vi "UI_(05A)_Set_Stop_State.vi"(3 "error in (no error)":errorcluster, 4 "Settings cluster in":T1={"Defaults"={"Default User"=0.0, "VISA Resource Name "=""}, "Recording and saving"={"Researcher name"="", "Name prefix"="", "Data post-processing"={"Filter type"=enum."Savitzky-Golay", "Length"=31, "Order"=3}, "Stop at"=0.0, "\"Stop at\" enabled"=FALSE, "Default save folder path"=path "", "Acquisition FPS"=enum."Max"}, "Geometry"={"Cage diameter, mm"=0, "Starting angle MIDFIELD"=0, "Starting angle BORDER"=0, "Radius, mm CENTER"=0, "Radius, mm MIDFIELD"=0, "N segments MIDFIELD"=0, "N segments BORDER"=0, "R-gap, mm"=0.0, "Bridge swap"=FALSE, "Bridge H. offset"=0.0, "Bridge V. offset"=0.0, "Twisted neck"=FALSE, "Alt. magn. orientation"=FALSE}, "IO parameters"={"IO general config."=0, "IO 1 configuration"=0, "IO 2 configuration"=0, "IO 3 configuration"=0, "IO 4 configuration"=0, "Activate ext. RS-232"=0, "IO inversion config."=0, "Sync capability"=1}, "Stimulus presets array"=[{"Event type"=0, "Dur., s"=0.0, "Stim., s"=0.0, "TTL out N"=1, "Set/Clear"=FALSE, "Stim. has been set"=FALSE}, {"Event type"=0, "Dur., s"=0.0, "Stim., s"=0.0, "TTL out N"=1, "Set/Clear"=FALSE, "Stim. has been set"=FALSE}, {"Event type"=0, "Dur., s"=0.0, "Stim., s"=0.0, "TTL out N"=1, "Set/Clear"=FALSE, "Stim. has been set"=FALSE}, {"Event type"=0, "Dur., s"=0.0, "Stim., s"=0.0, "TTL out N"=1, "Set/Clear"=FALSE, "Stim. has been set"=FALSE}, {"Event type"=0, "Dur., s"=0.0, "Stim., s"=0.0, "TTL out N"=1, "Set/Clear"=FALSE, "Stim. has been set"=FALSE}, {"Event type"=0, "Dur., s"=0.0, "Stim., s"=0.0, "TTL out N"=1, "Set/Clear"=FALSE, "Stim. has been set"=FALSE}, {"Event type"=0, "Dur., s"=0.0, "Stim., s"=0.0, "TTL out N"=1, "Set/Clear"=FALSE, "Stim. has been set"=FALSE}, {"Event type"=0, "Dur., s"=0.0, "Stim., s"=0.0, "TTL out N"=1, "Set/Clear"=FALSE, "Stim. has been set"=FALSE}, {"Event type"=0, "Dur., s"=0.0, "Stim., s"=0.0, "TTL out N"=1, "Set/Clear"=FALSE, "Stim. has been set"=FALSE}, {"Event type"=0, "Dur., s"=0.0, "Stim., s"=0.0, "TTL out N"=1, "Set/Clear"=FALSE, "Stim. has been set"=FALSE}, {"Event type"=0, "Dur., s"=0.0, "Stim., s"=0.0, "TTL out N"=1, "Set/Clear"=FALSE, "Stim. has been set"=FALSE}, {"Event type"=0, "Dur., s"=0.0, "Stim., s"=0.0, "TTL out N"=1, "Set/Clear"=FALSE, "Stim. has been set"=FALSE}, {"Event type"=0, "Dur., s"=0.0, "Stim., s"=0.0, "TTL out N"=1, "Set/Clear"=FALSE, "Stim. has been set"=FALSE}, {"Event type"=0, "Dur., s"=0.0, "Stim., s"=0.0, "TTL out N"=1, "Set/Clear"=FALSE, "Stim. has been set"=FALSE}], "Calibration parameters"={"Timing calibration sw/hw"=1.0, "True FPS"=80.0, "True frame time, s"=80.0, "Disp. calibration info"=[]}, "Settings loaded OK"=FALSE} {"Calibration parameters"."True frame time, s" format="%.10g"; "Calibration parameters"."Disp. calibration info"."Speed, µl per ms" format="%.3g"; "Calibration parameters"."True FPS" format="%.10g"; "Calibration parameters"."Timing calibration sw/hw" format="%.10g"; "Stimulus presets array"."Event type" items=["Stay for N seconds"]; "Stimulus presets array"."TTL out N" items=["1"=1, "2"=2, "1+2"=3]; "Recording and saving"."Data post-processing"."Order" min=3 max=11 step=2; "Recording and saving"."Data post-processing"."Length" min=5 max=301 step=2; "Geometry"."Cage diameter, mm" scale=0.0..340.0}, 5 "All references in":T11) -> (0 "error out":errorcluster, 1 "Settings cluster out":T1={"Defaults"={"Default User"=0.0, "VISA Resource Name "=""}, "Recording and saving"={"Researcher name"="", "Name prefix"="", "Data post-processing"={"Filter type"=enum."Savitzky-Golay", "Length"=31, "Order"=3}, "Stop at"=0.0, "\"Stop at\" enabled"=FALSE, "Default save folder path"=path "", "Acquisition FPS"=enum."Max"}, "Geometry"={"Cage diameter, mm"=0, "Starting angle MIDFIELD"=0, "Starting angle BORDER"=0, "Radius, mm CENTER"=0, "Radius, mm MIDFIELD"=0, "N segments MIDFIELD"=0, "N segments BORDER"=0, "R-gap, mm"=0.0, "Bridge swap"=FALSE, "Bridge H. offset"=0.0, "Bridge V. offset"=0.0, "Twisted neck"=FALSE, "Alt. magn. orientation"=FALSE}, "IO parameters"={"IO general config."=0, "IO 1 configuration"=0, "IO 2 configuration"=0, "IO 3 configuration"=0, "IO 4 configuration"=0, "Activate ext. RS-232"=0, "IO inversion config."=0, "Sync capability"=1}, "Stimulus presets array"=[{"Event type"=0, "Dur., s"=0.0, "Stim., s"=0.0, "TTL out N"=1, "Set/Clear"=FALSE, "Stim. has been set"=FALSE}, {"Event type"=0, "Dur., s"=0.0, "Stim., s"=0.0, "TTL out N"=1, "Set/Clear"=FALSE, "Stim. has been set"=FALSE}, {"Event type"=0, "Dur., s"=0.0, "Stim., s"=0.0, "TTL out N"=1, "Set/Clear"=FALSE, "Stim. has been set"=FALSE}, {"Event type"=0, "Dur., s"=0.0, "Stim., s"=0.0, "TTL out N"=1, "Set/Clear"=FALSE, "Stim. has been set"=FALSE}, {"Event type"=0, "Dur., s"=0.0, "Stim., s"=0.0, "TTL out N"=1, "Set/Clear"=FALSE, "Stim. has been set"=FALSE}, {"Event type"=0, "Dur., s"=0.0, "Stim., s"=0.0, "TTL out N"=1, "Set/Clear"=FALSE, "Stim. has been set"=FALSE}, {"Event type"=0, "Dur., s"=0.0, "Stim., s"=0.0, "TTL out N"=1, "Set/Clear"=FALSE, "Stim. has been set"=FALSE}, {"Event type"=0, "Dur., s"=0.0, "Stim., s"=0.0, "TTL out N"=1, "Set/Clear"=FALSE, "Stim. has been set"=FALSE}, {"Event type"=0, "Dur., s"=0.0, "Stim., s"=0.0, "TTL out N"=1, "Set/Clear"=FALSE, "Stim. has been set"=FALSE}, {"Event type"=0, "Dur., s"=0.0, "Stim., s"=0.0, "TTL out N"=1, "Set/Clear"=FALSE, "Stim. has been set"=FALSE}, {"Event type"=0, "Dur., s"=0.0, "Stim., s"=0.0, "TTL out N"=1, "Set/Clear"=FALSE, "Stim. has been set"=FALSE}, {"Event type"=0, "Dur., s"=0.0, "Stim., s"=0.0, "TTL out N"=1, "Set/Clear"=FALSE, "Stim. has been set"=FALSE}, {"Event type"=0, "Dur., s"=0.0, "Stim., s"=0.0, "TTL out N"=1, "Set/Clear"=FALSE, "Stim. has been set"=FALSE}, {"Event type"=0, "Dur., s"=0.0, "Stim., s"=0.0, "TTL out N"=1, "Set/Clear"=FALSE, "Stim. has been set"=FALSE}], "Calibration parameters"={"Timing calibration sw/hw"=1.0, "True FPS"=80.0, "True frame time, s"=80.0, "Disp. calibration info"=[]}, "Settings loaded OK"=FALSE} {"Calibration parameters"."True frame time, s" format="%.10g"; "Calibration parameters"."Disp. calibration info"."Speed, µl per ms" format="%.3g"; "Calibration parameters"."True FPS" format="%.10g"; "Calibration parameters"."Timing calibration sw/hw" format="%.10g"; "Stimulus presets array"."Event type" items=["Stay for N seconds"]; "Stimulus presets array"."TTL out N" items=["1"=1, "2"=2, "1+2"=3]; "Recording and saving"."Data post-processing"."Order" min=3 max=11 step=2; "Recording and saving"."Data post-processing"."Length" min=5 max=301 step=2; "Geometry"."Cage diameter, mm" scale=0.0..340.0}, 2 "All references out":T11)   [LabVIEW 2018, in "Tracker.lvlib"]
uses:
  Controls/CTL_All_References.ctl
  Controls/CTL_Controls_References.ctl
  Controls/CTL_Indicators_References.ctl
  Controls/CTL_Panes_and_VIs_References.ctl
  Controls/CTL_Histogram_Properties.ctl
  <vilib>/Utility/miscctls.llb/LVRangeTypeDef.ctl
  Controls/CTL_Settings_cluster.ctl
  Controls/CTL_Filter_selector.ctl
  Controls/CTL_Acquisition_speed_selector.ctl
  Controls/CTL_Segmented_plot_parameters.ctl
  Controls/CTL_IO_params_cluster.ctl
  Controls/CTL_Single_stimulus_setting.ctl
  Controls/CTL_Calibration_parameters.ctl
  Controls/CTL_Dispenser_calibration_info.ctl
  <vilib>/Utility/error.llb/Error Cluster From Error Code.vi
  <vilib>/ErrorRing/Error Ring.xnode
  Tracker.lvlib
panel:
  in  "Histogram initialization cluster":T9={"X Scale.Range"={"Minimum"=0.0, "Maximum"=13.0, "Increment"=1.0, "Minor Increment"=1.0, "Start"=0.0}, "Caption.Text"="Zone preference (normalized)", "X Scale.Offset and Multiplier:Multiplier"=1.0, "X Scale.Offset and Multiplier:Offset"=0.0, "X Scale.Scale Fit"=2, "X Scale.Display Format:Precision"=0, "Y Scale.Mapping Mode"=0, "Zones preference empty initialized array"=[0, 0, 0, 0, 0, 0, 0, 0, 0, 0, 0, 0, 0, 0], "Plot.Fill/Point Color"=15790320}
  out "Panes references":T14
  out "Controls references params":string[][](array[string])
  out "Indicators references params":string[][](array[string])
  out "Indicators references":T13
  out "Controls references":T12
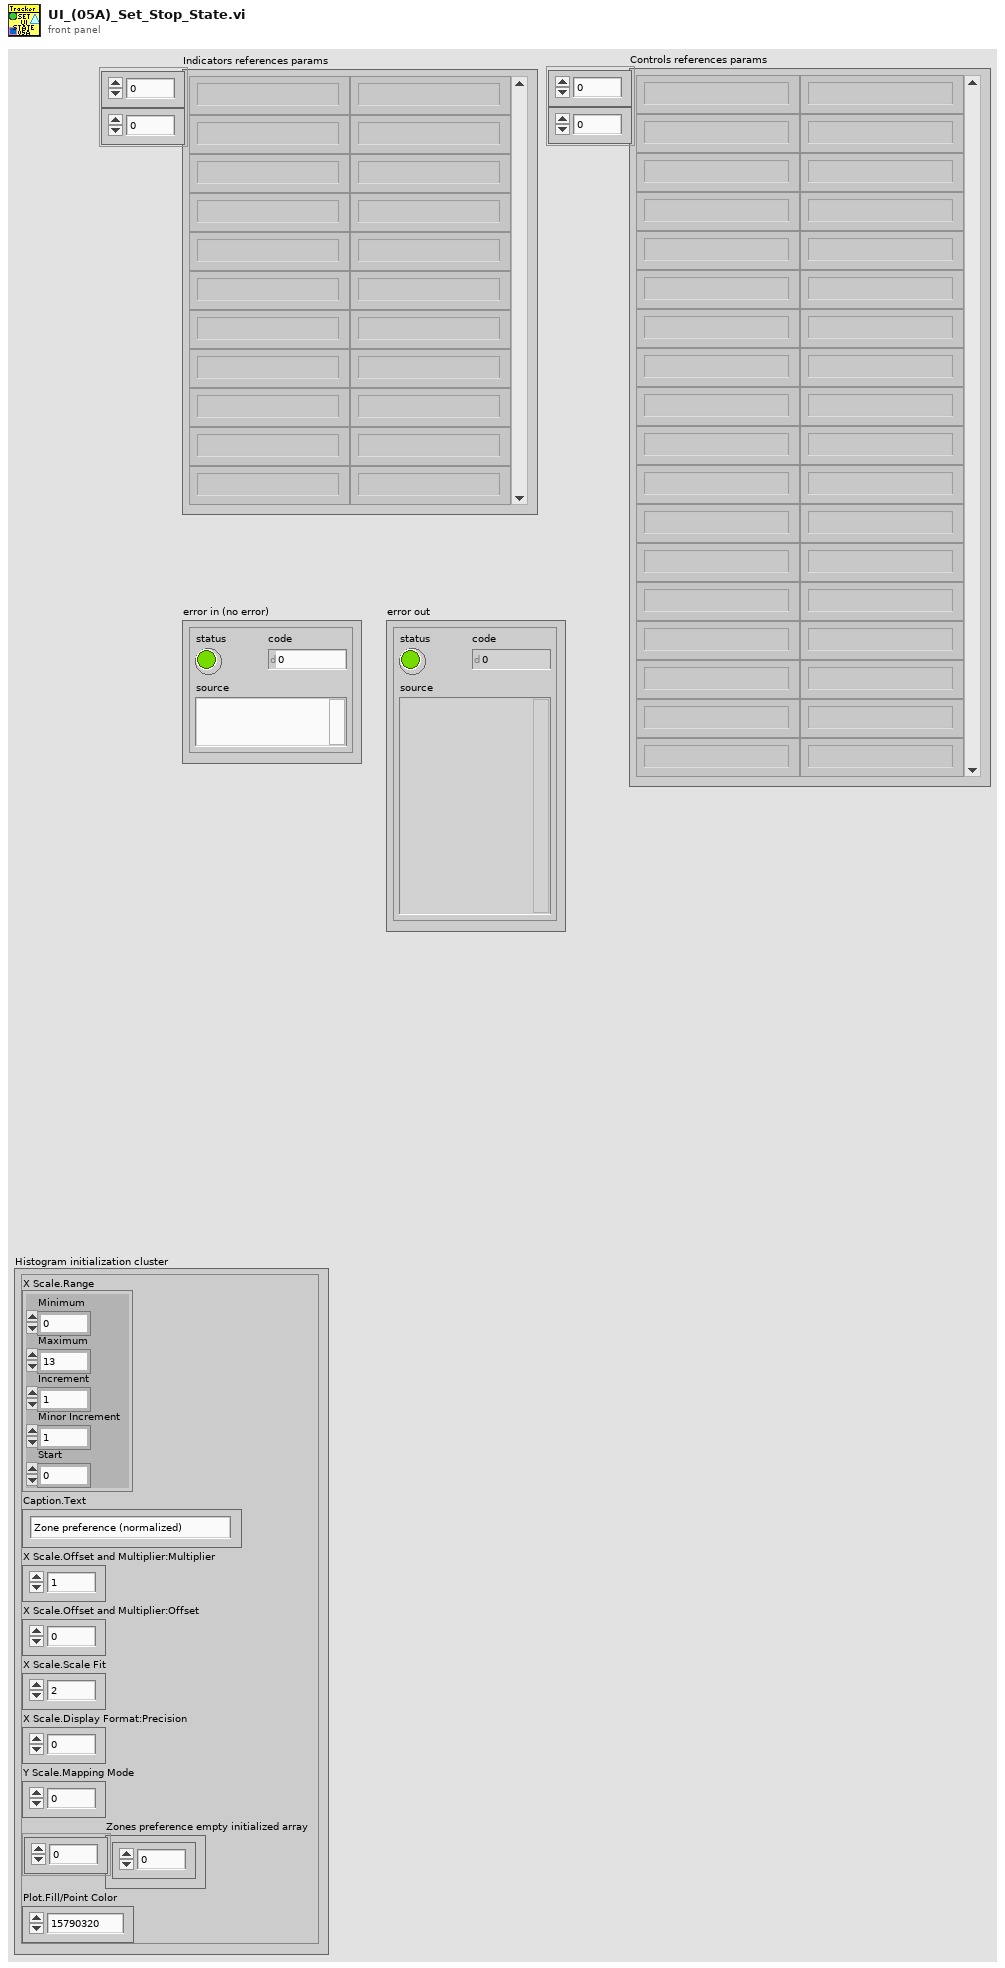
[diagram p1: front panel]
types:
  T1 = typedef "Tracker.lvlib/CTL_Settings_cluster.ctl" = cluster{"Defaults":cluster{"Default User":dbl, "VISA Resource Name ":string}, "Recording and saving":cluster{"Researcher name":string, "Name prefix":string, "Data post-processing":T2, "Stop at":dbl, "\"Stop at\" enabled":bool, "Default save folder path":path, "Acquisition FPS":T3}, "Geometry":T4, "IO parameters":T5, "Stimulus presets array":T6[], "Calibration parameters":T7, "Settings loaded OK":bool}
  T2 = typedef "Tracker.lvlib/CTL_Filter_selector.ctl" = cluster{"Filter type":enum16{"None", "Savitzky-Golay"}, "Length":i32, "Order":i32}
  T3 = typedef "Tracker.lvlib/CTL_Acquisition_speed_selector.ctl" = enum16{"Max", "Optimal", "Eco"}
  T4 = typedef "Tracker.lvlib/CTL_Segmented_plot_parameters.ctl" = cluster{"Cage diameter, mm":u16, "Starting angle MIDFIELD":i16, "Starting angle BORDER":i16, "Radius, mm CENTER":u16, "Radius, mm MIDFIELD":u16, "N segments MIDFIELD":u8, "N segments BORDER":u8, "R-gap, mm":sgl, "Bridge swap":bool, "Bridge H. offset":sgl, "Bridge V. offset":sgl, "Twisted neck":bool, "Alt. magn. orientation":bool}
  T5 = typedef "Tracker.lvlib/CTL_IO_params_cluster.ctl" = cluster{"IO general config.":u16, "IO 1 configuration":u16, "IO 2 configuration":u16, "IO 3 configuration":u16, "IO 4 configuration":u16, "Activate ext. RS-232":u16, "IO inversion config.":u16, "Sync capability":u8}
  T6 = typedef "Tracker.lvlib/CTL_Single_stimulus_setting.ctl" = cluster{"Event type":u16, "Dur., s":sgl, "Stim., s":sgl, "TTL out N":u16, "Set/Clear":bool, "Stim. has been set":bool}
  T7 = typedef "Tracker.lvlib/CTL_Calibration_parameters.ctl" = cluster{"Timing calibration sw/hw":dbl, "True FPS":dbl, "True frame time, s":dbl, "Disp. calibration info":T8}
  T8 = typedef "Tracker.lvlib/CTL_Dispenser_calibration_info.ctl" = cluster{"Channel":u8, "Speed, µl per ms":dbl}[]
  T9 = typedef "Tracker.lvlib/CTL_Histogram_Properties.ctl" = cluster{"X Scale.Range":T10, "Caption.Text":string, "X Scale.Offset and Multiplier:Multiplier":dbl, "X Scale.Offset and Multiplier:Offset":dbl, "X Scale.Scale Fit":u8, "X Scale.Display Format:Precision":u8, "Y Scale.Mapping Mode":u8, "Zones preference empty initialized array":i32[], "Plot.Fill/Point Color":u32}
  T10 = typedef "LVRangeTypeDef.ctl" = cluster{"Minimum":dbl, "Maximum":dbl, "Increment":dbl, "Minor Increment":dbl, "Start":dbl}
  T11 = typedef "Tracker.lvlib/CTL_All_References.ctl" = cluster{"Controls references":T12, "Indicators references":T13, "Service references":T14}
  T12 = typedef "Tracker.lvlib/CTL_Controls_References.ctl" = cluster{"Check HW connection":refnum<vi>, "Start Tracking button":refnum<vi>, "Reset zones":refnum<vi>, "Reset stimuli":refnum<vi>, "Record/Stop":refnum<vi>, "Reset barplot":refnum<vi>, "Multiplyer of chart RX":refnum<vi>, "Show zones":refnum<vi>, "Show magnets":refnum<vi>, "Show heatmap":refnum<vi>, "Show full track":refnum<vi>, "Open File":refnum<vi>, "Play/Pause":refnum<vi>, "Trace, s":refnum<vi>, "Playback speed":refnum<vi>, "Timeline":refnum<vi>, "By Zone stim. setup":refnum<vi>, "Set, Rec and Analyse Tab":refnum<vi>, "Cage radial segmentation":refnum<vi>, "Set IO config":refnum<vi>, "Rainbow (time)":refnum<vi>, "Rainbow (speed)":refnum<vi>}
  T13 = typedef "Tracker.lvlib/CTL_Indicators_References.ctl" = cluster{"HW info":refnum<vi>, "Port":refnum<vi>, "Ready":refnum<vi>, "IO status indicator":refnum<vi>, "Current Time":refnum<vi>, "Record timestamp":refnum<vi>, "Mouse speed":refnum<vi>, "Mouse speed, mm/s":refnum<vi>, "Running, perc. of time":refnum<vi>, "Histograms":refnum<vi>, "Cage size":refnum<vi>}
  T14 = typedef "Tracker.lvlib/CTL_Panes_and_VIs_References.ctl" = cluster{"Pane":refnum<vi>, "This VI":refnum<vi>, "Menu":refnum<k9>}
  T15 = enum8{"Enabled", "Disabled", "Disabled and Grayed Out"}
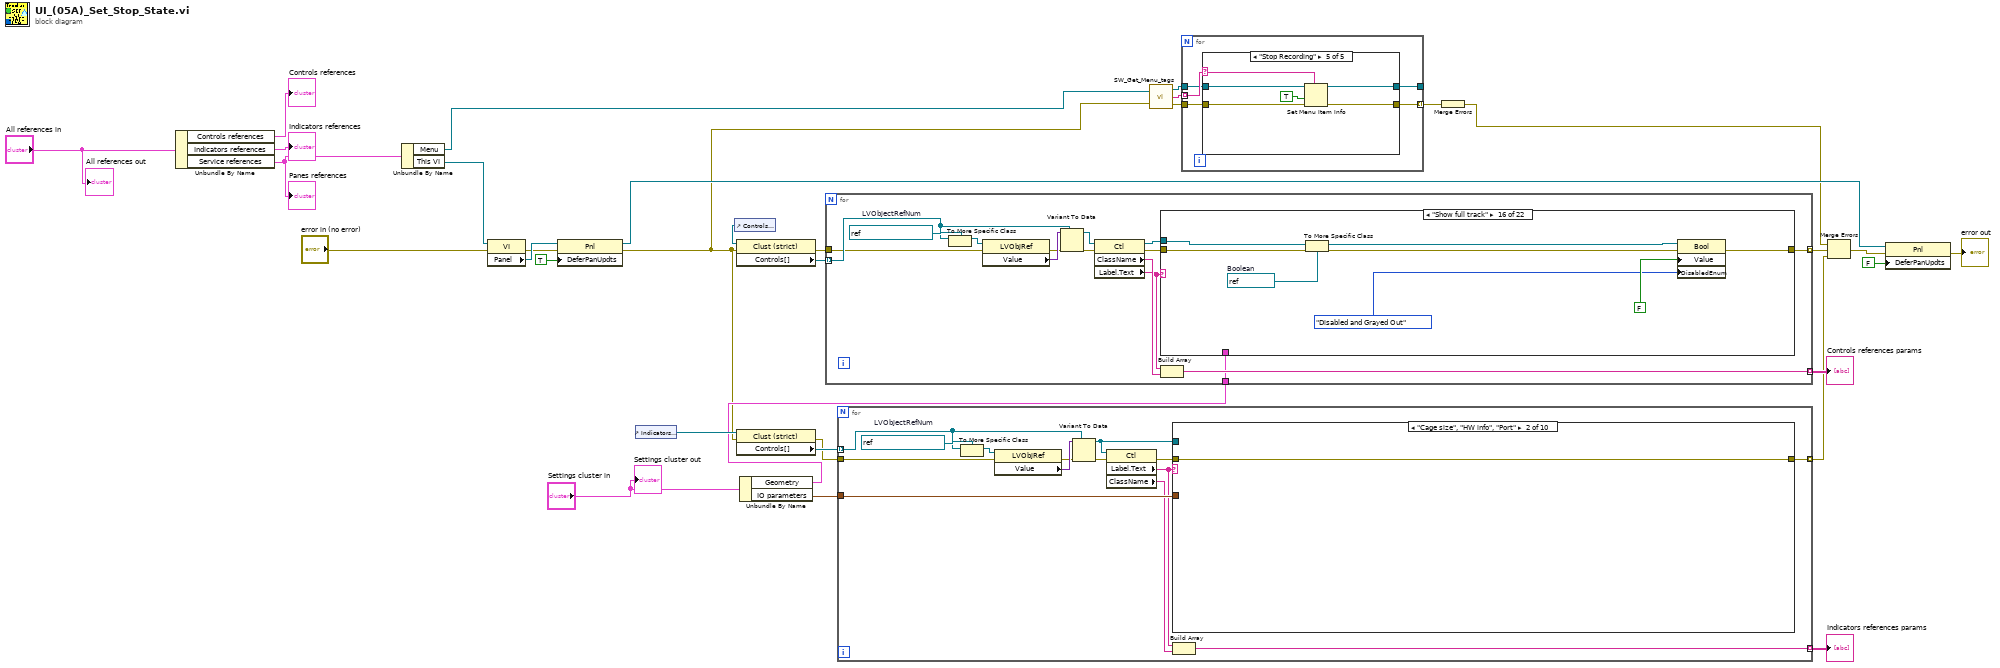
[diagram p0: block diagram]
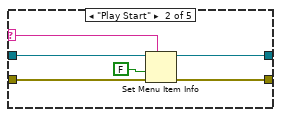
[diagram p3: hidden frame]
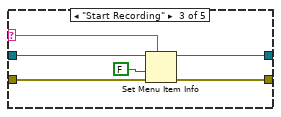
[diagram p4: hidden frame]
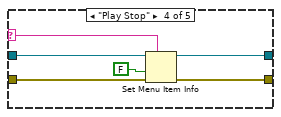
[diagram p5: hidden frame]
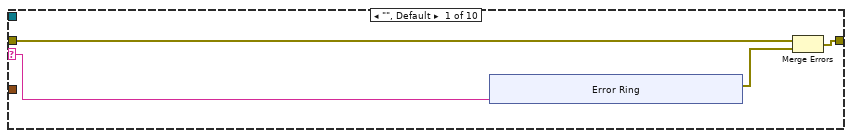
[diagram p6: hidden frame]
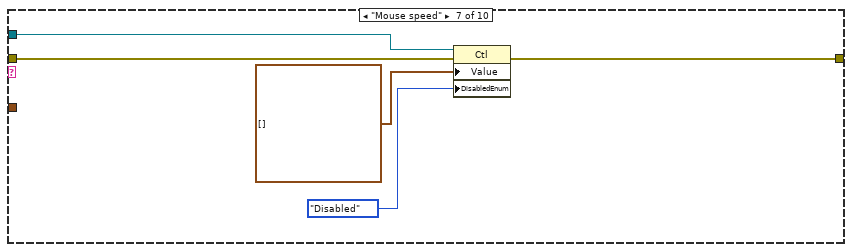
[diagram p11: hidden frame]
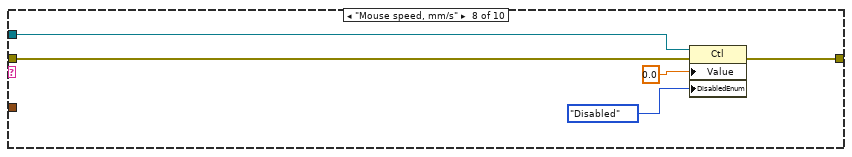
[diagram p12: hidden frame]
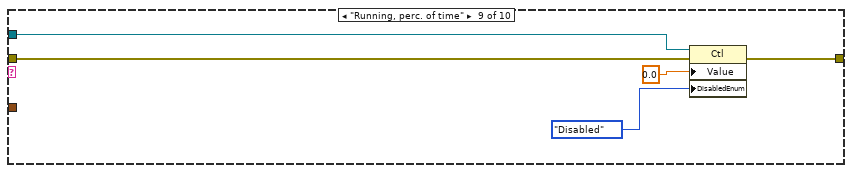
[diagram p13: hidden frame]
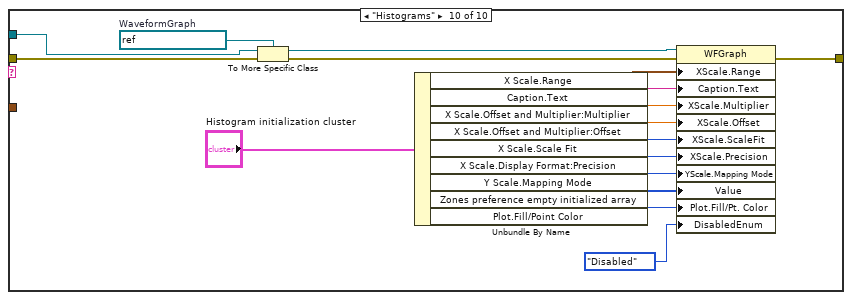
[diagram p14: hidden frame]
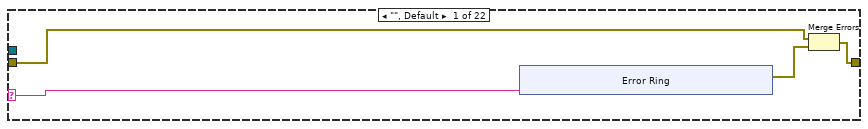
[diagram p15: hidden frame]
diagram:
  n1 = Unbundle By Name("All references in") -> ("Controls references"=→"Controls references":T12, "Indicators references"=→"Indicators references":T13, "Service references"=w24:T14)
  "Panes references" <- w24
  n2 = Unbundle By Name(w24) -> ("Menu"=w3:refnum<k9>, "This VI"=w21:refnum<vi>)
  n3 = property class="VI"(reference=w21, error in="error in (no error)") -> (error out=w14:errorcluster, "Panel"=w23:refnum<vi>)  [unwired: 1 out]
  n4 = property class="Pnl"(reference=w23, error in=w14, "DeferPanUpdts"=TRUE ("Defer Panel Updates")) -> (reference out=w15:refnum<vi>, error out=w2:errorcluster)
  n5 = control-ref of="Indicators references"() -> (w27:refnum<vi>)
  n6 = control-ref of="Controls references"() -> (w29:refnum<vi>)
  n7 = property class="Clust (strict)"(reference=w29, error in=w2) -> (error out=w20:errorcluster, "Controls[]"=w30:refnum<vi>[])  [unwired: 1 out]
  n8 = property class="Clust (strict)"(reference=w27, error in=w2) -> (error out=w19:errorcluster, "Controls[]"=w28:refnum<vi>[])  [unwired: 1 out]
  n9 = Unbundle By Name("Settings cluster in") -> ("Geometry"=w8:T4, "IO parameters"=w10:T5)
  n10 = for {
    tunnel: w30 -> [w45] mode=indexing
    tunnel: [w42] -> w25 mode=indexing
    tunnel: w20 -> [w41]
    tunnel: [w37] -> w12 mode=indexing
    tunnel: w8 -> [w34]
    w47 = refnum<vi> refnum  # LVObjectRefNum
    n11 = To More Specific Class(target class=w47, reference=w45) -> (specific class reference=w48:refnum<vi>)  [unwired: 1 in, 1 out]
    n12 = property class="LVObjRef"(reference=w48, error in=w41) -> (error out=w40:errorcluster, "Value"=w46:variant)  [unwired: 1 out]
    n13 = Variant To Data(error in=w40, type=w45, Variant=w46) -> (data=w44:refnum<vi>, error out=w39:errorcluster)
    n14 = property class="Ctl"(reference=w44, error in=w39) -> (reference out=w35:refnum<vi>, error out=w36:errorcluster, "ClassName"=w43:string, "Label.Text"=w38:string)
    n15 = case shown="\"Show full track\"" w38 {
      selector: w38 -> [w49 _ _ _ _ _ _ _ _ _ _ _ _ _ _ _ _ _ _ _ _ _]
      tunnel: [w51 w60 w61 w62 w63 w64 w65 w66 w67 w70 w78 w86 w92 w93 w102 w110 w116 w117 w126 w134 w142 w148] -> w37
      tunnel: w36 -> [w52 w60 w61 w62 w63 w64 w65 w66 w67 w72 w80 w88 w92 w95 w104 w112 w116 w118 w128 w136 w144 w148]
      tunnel: w35 -> [_ _ _ _ _ _ _ _ _ w75 w83 w91 _ w94 w107 w115 _ w119 w131 w139 w147 _]
      tunnel: w34 -> [_ _ _ _ _ _ _ _ _ _ _ _ _ _ _ _ _ _ _ _ _ _]
      frame "", Default {
        n16 = xnode "Error Ring"("parameter 0"=w49) -> ("error out"=w50:errorcluster)
        n17 = Merge Errors(w52, w50) -> (w51:errorcluster)
      }
      frame "Cage radial segmentation" {
      }
      frame "Set/Rec and Analyse Tab" {
      }
      frame "Check HW connection" {
      }
      frame "Save settings" {
      }
      frame "Set IO config" {
      }
      frame "Reset zones" {
      }
      frame "Reset stimuli" {
      }
      frame "Record/Stop" {
      }
      frame "Reset barplot" {
        w74 = refnum<vi> refnum  # Boolean
        n18 = To More Specific Class(target class=w74, reference=w75, error in=w72) -> (specific class reference=w73:refnum<vi>, error out=w71:errorcluster)
        n19 = property class="Bool"(reference=w73, error in=w71, "Value"=FALSE, "DisabledEnum"=T15."Enabled" ("Disabled")) -> (error out=w70:errorcluster)  [unwired: 1 out]
      }
      frame "Multiplyer of chart RX" {
        w82 = refnum<vi> refnum  # Slide
        n20 = To More Specific Class(target class=w82, reference=w83, error in=w80) -> (specific class reference=w81:refnum<vi>, error out=w79:errorcluster)
        n21 = property class="Slide"(reference=w81, error in=w79, "Value"=u8 1, "DisabledEnum"=T15."Enabled" ("Disabled")) -> (error out=w78:errorcluster)  [unwired: 1 out]
      }
      frame "Show zones" {
        w90 = refnum<vi> refnum  # Boolean
        n22 = To More Specific Class(target class=w90, reference=w91, error in=w88) -> (specific class reference=w89:refnum<vi>, error out=w87:errorcluster)
        n23 = property class="Bool"(reference=w89, error in=w87, "Value"=TRUE, "DisabledEnum"=T15."Enabled" ("Disabled")) -> (error out=w86:errorcluster)  [unwired: 1 out]
      }
      frame "Show magnets" {
      }
      frame "Rainbow (speed)", "Rainbow (time)" {
        w96 = refnum<vi> refnum  # Boolean
        n24 = To More Specific Class(target class=w96, reference=w94, error in=w95) -> (specific class reference=w98:refnum<vi>, error out=w99:errorcluster)
        n25 = property class="Bool"(reference=w98, error in=w99, "DisabledEnum"=T15."Enabled" ("Disabled")) -> (error out=w93:errorcluster)  [unwired: 1 out]
      }
      frame "Show heatmap" {
        w106 = refnum<vi> refnum  # Boolean
        n26 = To More Specific Class(target class=w106, reference=w107, error in=w104) -> (specific class reference=w105:refnum<vi>, error out=w103:errorcluster)
        n27 = property class="Bool"(reference=w105, error in=w103, "Value"=FALSE, "DisabledEnum"=T15."Disabled and Grayed Out" ("Disabled")) -> (error out=w102:errorcluster)  [unwired: 1 out]
      }
      frame "Show full track" {
        w114 = refnum<vi> refnum  # Boolean
        n28 = To More Specific Class(target class=w114, reference=w115, error in=w112) -> (specific class reference=w113:refnum<vi>, error out=w111:errorcluster)
        n29 = property class="Bool"(reference=w113, error in=w111, "Value"=FALSE, "DisabledEnum"=T15."Disabled and Grayed Out" ("Disabled")) -> (error out=w110:errorcluster)  [unwired: 1 out]
      }
      frame "Open File" {
      }
      frame "Play/Pause" {
        w120 = refnum<vi> refnum  # Boolean
        n30 = To More Specific Class(target class=w120, reference=w119, error in=w118) -> (specific class reference=w123:refnum<vi>, error out=w122:errorcluster)
        n31 = property class="Bool"(reference=w123, error in=w122, "DisabledEnum"=T15."Disabled and Grayed Out" ("Disabled")) -> (error out=w117:errorcluster)  [unwired: 1 out]
      }
      frame "Trace, s" {
        w130 = refnum<vi> refnum  # Slide
        n32 = To More Specific Class(target class=w130, reference=w131, error in=w128) -> (specific class reference=w129:refnum<vi>, error out=w127:errorcluster)
        n33 = property class="Slide"(reference=w129, error in=w127, "Value"=u8 5, "DisabledEnum"=T15."Enabled" ("Disabled")) -> (error out=w126:errorcluster)  [unwired: 1 out]
      }
      frame "Playback speed" {
        w138 = refnum<vi> refnum  # Ring
        n34 = To More Specific Class(target class=w138, reference=w139, error in=w136) -> (specific class reference=w137:refnum<vi>, error out=w135:errorcluster)
        n35 = property class="Ring"(reference=w137, error in=w135, "Value"=u8 3, "DisabledEnum"=T15."Disabled and Grayed Out" ("Disabled")) -> (error out=w134:errorcluster)  [unwired: 1 out]
      }
      frame "Timeline" {
        w146 = refnum<vi> refnum  # Slide
        n36 = To More Specific Class(target class=w146, reference=w147, error in=w144) -> (specific class reference=w145:refnum<vi>, error out=w143:errorcluster)
        n37 = property class="Slide"(reference=w145, error in=w143, "Value"=u8 5, "DisabledEnum"=T15."Disabled and Grayed Out" ("Disabled")) -> (error out=w142:errorcluster)  [unwired: 1 out]
      }
      frame "By Zone stim. setup" {
      }
    }
    n38 = Build Array(w38, w43) -> (w42:string[])
  }
  "Controls references params" <- w25
  n39 = for {
    tunnel: w28 -> [w159] mode=indexing
    tunnel: [w149] -> w26 mode=indexing
    tunnel: w19 -> [w157]
    tunnel: [w153] -> w18 mode=indexing
    tunnel: w10 -> [w152]
    w161 = refnum<vi> refnum  # LVObjectRefNum
    n40 = To More Specific Class(target class=w161, reference=w159) -> (specific class reference=w162:refnum<vi>)  [unwired: 1 in, 1 out]
    n41 = property class="LVObjRef"(reference=w162, error in=w157) -> (error out=w156:errorcluster, "Value"=w160:variant)  [unwired: 1 out]
    n42 = Variant To Data(error in=w156, type=w159, Variant=w160) -> (data=w158:refnum<vi>, error out=w155:errorcluster)
    n43 = property class="Ctl"(reference=w158, error in=w155) -> (error out=w154:errorcluster, "Label.Text"=w151:string, "ClassName"=w150:string)  [unwired: 1 out]
    n44 = case shown="\"Cage size\", \"HW info\", \"Port\"" w151 {
      selector: w151 -> [w163 _ _ _ _ _ _ _ _ _]
      tunnel: w158 -> [_ _ _ _ _ _ w183 w188 w193 w210]
      tunnel: w154 -> [w166 w174 w175 w176 w177 w178 w182 w187 w192 w196]
      tunnel: [w165 w174 w175 w176 w177 w178 w181 w186 w191 w209] -> w153
      tunnel: w152 -> [_ _ _ _ _ _ _ _ _ _]
      frame "", Default {
        n45 = xnode "Error Ring"("parameter 0"=w163) -> ("error out"=w164:errorcluster)
        n46 = Merge Errors(w166, w164) -> (w165:errorcluster)
      }
      frame "Cage size", "HW info", "Port" {
      }
      frame "Ready" {
      }
      frame "IO status indicator" {
      }
      frame "Current Time" {
      }
      frame "Record timestamp" {
      }
      frame "Mouse speed" {
        n47 = property class="Ctl"(reference=w183, error in=w182, "Value"=waveform(dbl)[] [] ("History Data"), "DisabledEnum"=T15."Disabled" ("Disabled")) -> (error out=w181:errorcluster)  [unwired: 1 out]
      }
      frame "Mouse speed, mm/s" {
        n48 = property class="Ctl"(reference=w188, error in=w187, "Value"=0.0, "DisabledEnum"=T15."Disabled" ("Disabled")) -> (error out=w186:errorcluster)  [unwired: 1 out]
      }
      frame "Running, perc. of time" {
        n49 = property class="Ctl"(reference=w193, error in=w192, "Value"=0.0, "DisabledEnum"=T15."Disabled" ("Disabled")) -> (error out=w191:errorcluster)  [unwired: 1 out]
      }
      frame "Histograms" {
        w207 = refnum<vi> refnum  # WaveformGraph
        n50 = To More Specific Class(target class=w207, reference=w210, error in=w196) -> (specific class reference=w208:refnum<vi>, error out=w195:errorcluster)
        n51 = Unbundle By Name("Histogram initialization cluster") -> ("X Scale.Range"=w205:T10, "Caption.Text"=w204:string, "X Scale.Offset and Multiplier:Multiplier"=w203:dbl, "X Scale.Offset and Multiplier:Offset"=w202:dbl, "X Scale.Scale Fit"=w201:u8, "X Scale.Display Format:Precision"=w200:u8, "Y Scale.Mapping Mode"=w199:u8, "Zones preference empty initialized array"=w198:i32[], "Plot.Fill/Point Color"=w197:u32)
        n52 = property class="WFGraph"(reference=w208, error in=w195, "XScale.Range"=w205, "Caption.Text"=w204, "XScale.Multiplier"=w203, "XScale.Offset"=w202, "XScale.ScaleFit"=w201, "XScale.Precision"=w200, "YScale.Mapping Mode"=w199, "Value"=w198, "Plot.Fill/Pt. Color"=w197, "DisabledEnum"=T15."Disabled" ("Disabled")) -> (error out=w209:errorcluster)  [unwired: 1 out]
      }
    }
    n53 = Build Array(w151, w150) -> (w149:string[])
  }
  "Indicators references params" <- w26
  n54 = call "SW_Get_Menu_tags.vi"("Menu ref in"=w3, "error in (no error)"=w2) -> ("Menu ref out"=w5:refnum<k9>, "(Sub)menu tags"=w7:string[], "error out"=w6:errorcluster)
  n55 = for {
    tunnel: w7 -> [w215] mode=indexing
    tunnel: w6 -> [w214]
    tunnel: [w213] -> w4 mode=indexing
    tunnel: [w212] -> _
    tunnel: w5 -> [w211]
    n56 = case shown="\"Stop Recording\"" w215 {
      selector: w215 -> [_ w223 w229 w235 w241]
      tunnel: w214 -> [w217 w221 w227 w233 w239]
      tunnel: [w217 w220 w226 w232 w238] -> w213
      tunnel: [w216 w219 w225 w231 w237] -> w212
      tunnel: w211 -> [w216 w218 w224 w230 w236]
      frame "", Default {
      }
      frame "Play Start" {
        n57 = Set Menu Item Info(7:w223, 8:w221, 9:FALSE ("enabled"), 11:w218) -> (0:w220:errorcluster, 3:w219:refnum<k9>)  [unwired: 3 in]
      }
      frame "Start Recording" {
        n58 = Set Menu Item Info(7:w229, 8:w227, 9:FALSE ("enabled"), 11:w224) -> (0:w226:errorcluster, 3:w225:refnum<k9>)  [unwired: 3 in]
      }
      frame "Play Stop" {
        n59 = Set Menu Item Info(7:w235, 8:w233, 9:FALSE ("enabled"), 11:w230) -> (0:w232:errorcluster, 3:w231:refnum<k9>)  [unwired: 3 in]
      }
      frame "Stop Recording" {
        n60 = Set Menu Item Info(7:w241, 8:w239, 9:TRUE ("enabled"), 11:w236) -> (0:w238:errorcluster, 3:w237:refnum<k9>)  [unwired: 3 in]
      }
    }
  }
  n61 = Merge Errors(w4) -> (w1:errorcluster)
  n62 = Merge Errors(w1, w12, w18) -> (w17:errorcluster)
  n63 = property class="Pnl"(reference=w15, error in=w17, "DeferPanUpdts"=FALSE ("Defer Panel Updates")) -> (error out=→"error out":errorcluster)  [unwired: 1 out]
  "All references out" <- "All references in"
  "Settings cluster out" <- "Settings cluster in"
